vi "TPIBuildMessage.vi"(10 "Command":string="ªU\u0000\u0002\b\u0001ô") -> (2 "Message":string)   [LabVIEW 2020]
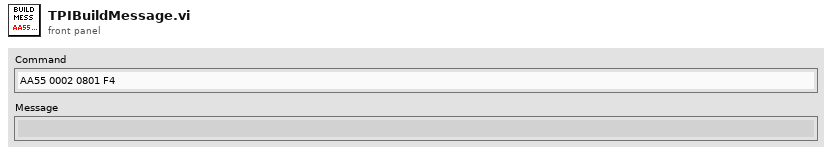
[diagram p1: front panel]
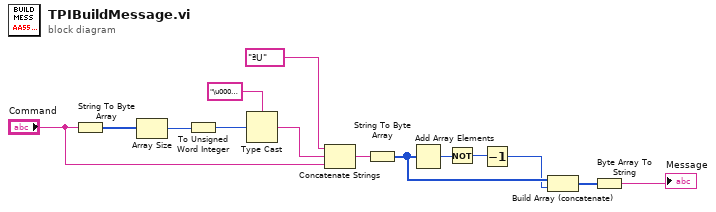
[diagram p0: block diagram]
diagram:
  n1 = String To Byte Array(string="Command") -> (unsigned byte array=w14:u8[])
  n2 = Array Size(array=w14) -> (size(s)=w6:i32)
  n3 = To Unsigned Word Integer(number=w6) -> (unsigned 16bit integer=w5:u16)
  n4 = Type Cast(type="\u0000\u0000" ("string"), x=w5) -> (*(type *) &x=w2:string)
  n5 = Concatenate Strings("ªU" ("string"), w2, "Command") -> (w13:string)
  n6 = String To Byte Array(string=w13) -> (unsigned byte array=w11:u8[])
  n7 = Add Array Elements(numeric array=w11) -> (sum=w12:u8)
  n8 = Not(x=w12) -> (.not. x?=w8:u8)
  n9 = Decrement(x=w8) -> (x-1=w7:u8)
  n10 = Build Array (concatenate)(w11, w7) -> (w10:u8[])
  n11 = Byte Array To String(unsigned byte array=w10) -> (string=→"Message":string)
